vi "AInScFg.VI"(3 "BoardNum":u32, 4 "LowChan":i32, 5 "InterChannel Delay":sgl=-1.0 format="%.2f", 6 "HighChan":i32, 7 "Options":i32, 8 "Range":i32(ring)=2 items=["Not Programmable"=0, "+- 20 V"=27, "+- 10 V"=1, "+- 5 V"=2, "+- 4 V"=28, "+- 2.5 V"=3, "+- 2 V"=29, "+- 1.67 V"=4, "+- 1.25 V"=5, "+- 1 V"=6, "+- .625 V"=7, "+- .5 V"=8, "+- .25 V"=30, "+- .2 V"=31, "+- .1 V"=9, "+- .05 V"=10, "+- .01 V"=11, "+- .005 V"=12, "0 - 10 V"=13, "0 - 5 V"=14, "0 - 4 V"=36, "0 - 2.5 V"=15, "0 - 2 V"=16, "0 - 1.67 V"=17, "0 - 1.25 V"=18, "0 - 1 V"=19, "0 - .5 V"=32, "0 - .25 V"=33, "0 - .2 V"=34, "0 - .1 V"=20, "0 - .02 V"=35, "0 - .01 V"=21, "4 - 20 mA"=22, "2 - 10 mA"=23, "1 - 5 mA"=24, ".5 - 2.5 mA"=25, "0 - 20 mA"=26], 9 "Rate":i32, 10 "Count":i32) -> (0 "ErrCode":i32, 1 "ADData":u16[](array[numeric]), 2 "Rate":i32)   [LabVIEW 2019, in "DAQ_Engine.lvclass"]
doc: "Developed by Kevin Thompson\nkevin@thompsonengineering.net\n\nCopyright 2020\nThompson Engineering, LLC\nScans a range of AD channels in the foreground and stores the samples in an array. This VI will not return control to your program until the requested data has been collected or a fatal error occurs."
uses:
  DAQ_Engine.lvclass
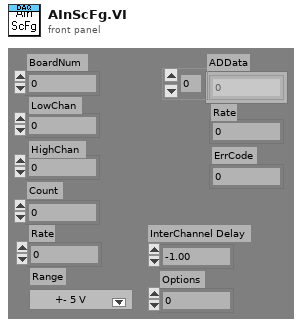
[diagram p1: front panel]
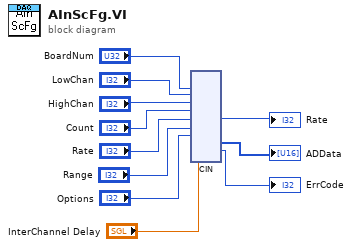
[diagram p0: block diagram]
diagram:
  n1 = cin("BoardNum", "LowChan", "HighChan", "Count", "Rate", "Range", "Options", "InterChannel Delay") -> (→"Rate":i32, →"ADData":u16[], →"ErrCode":i32)  [unwired: 9 in]
